vi "Start Logger.vi"(8 "error in (no error)":errorcluster, 11 "Data Processor Module in":refnum<class "Data Processor Module.lvclass">) -> (0 "error out":errorcluster, 3 "Data Processor Module out":refnum<class "Data Processor Module.lvclass">)   [LabVIEW 2020, in "VolatusData.lvlib" / "Data Processor Module.lvclass"]
uses:
  Data Processor Module.lvclass
  C:/dev/lv20CE/relink/lv-volatus/Volatus/Module/Module.lvclass
  VolatusConfig/VolatusConfigElement/VolatusConfigElement.lvclass
  Data Processor Module.lvclass/Data Processor Module.ctl
  Volatus/Module/Module.lvclass/Module.ctl
  VolatusConfig/VolatusConfigElement/VolatusConfigElement.lvclass/VolatusConfigElement.ctl
  Data Logger Module/Data Logger Module.lvclass
  Volatus/Module/Module.lvclass
  lv-cdm/CDM-Config/Config Element/Config Element.lvclass
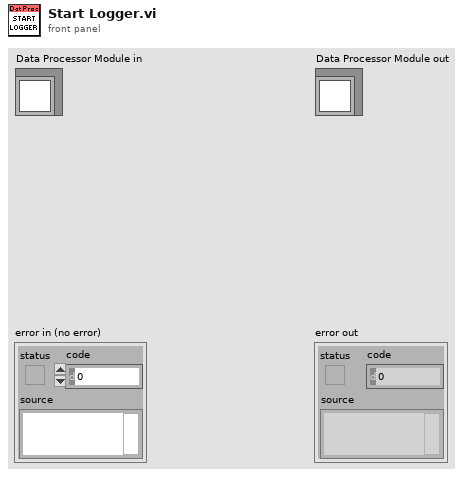
[diagram p1: front panel]
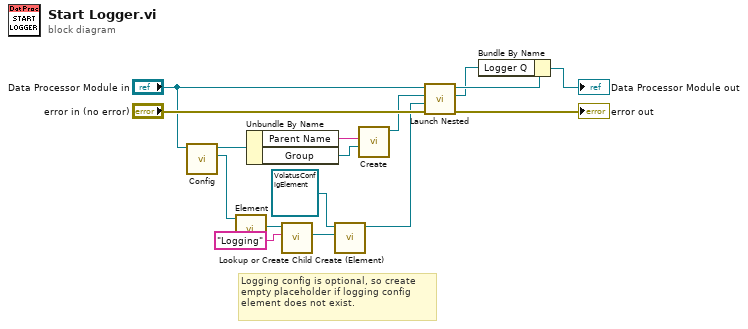
[diagram p0: block diagram]
diagram:
  # "Logging config is optional, so create empty placeholder if logging config element does not exist."
  n1 = call "Config.vi"("Module in"="Data Processor Module in") -> ("Config"=w6:refnum<class "VolatusConfigElement.lvclass">, "Module out"=w7:refnum<class "Data Processor Module.lvclass">)  [unwired: 9 in]
  n2 = call "Element.vi"("VolatusConfigElement in"=w6) -> ("Element"=w5:refnum<class "Config Element.lvclass">)  [unwired: 9 in, 1 out]
  n3 = Unbundle By Name(w7) -> ("Parent Name"=w15:string, "Group"=w9:refnum<class "Group.lvclass">)
  n4 = call "Lookup or Create Child.vi"("Name"="Logging", "Config Element in"=w5) -> ("Child"=w3:refnum<class "Config Element.lvclass">)  [unwired: 6 in, 3 out]
  n5 = call "Create (Element).vi"("Element"=w3, "VolatusConfigElement in"=refnum<class "VolatusConfigElement.lvclass"> refnum ("Config Element")) -> ("VolatusConfigElement out"=w1:refnum<class "VolatusConfigElement.lvclass">)  [unwired: 8 in, 1 out]
  n6 = call "Create.vi"("Group"=w9, "Parent Name"=w15) -> ("Data Logger Module out"=w12:refnum<class "Data Logger Module.lvclass">)  [unwired: 8 in, 1 out]
  n7 = call "Launch Nested.vi"("error in (no error)"="error in (no error)", "Config Element"=w1, "Nested Module"=w12, "Parent in"="Data Processor Module in") -> ("error out"=→"error out":errorcluster, "MessageQ"=w10:refnum<class "MessageQ.lvclass">, "Parent out"=w13:refnum<class "Data Processor Module.lvclass">)  [unwired: 5 in]
  n8 = Bundle By Name(cluster=w13, "Logger Q"=w10) -> (→"Data Processor Module out":refnum<class "Data Processor Module.lvclass">)
